vi "FTW-Actor-Destroy.vi"(0 "FTW Actor Instance":refnum<class "FTW-ActorInstance.lvclass">, 11 "error in":errorcluster) -> (15 "error out":errorcluster)   [LabVIEW 2012, in "FTW-Actor.lvlib" / "FTW-ActorInstance.lvclass"]
uses:
  FTW-ActorInstance.lvclass
  JobSequencer/FTW-JobSequencer.lvclass
  EventLogger/FTW-Logger.lvclass
  Endpoint/FTW-Endpoint.lvclass
panel:
  # "Inputs"
  # "Outputs"
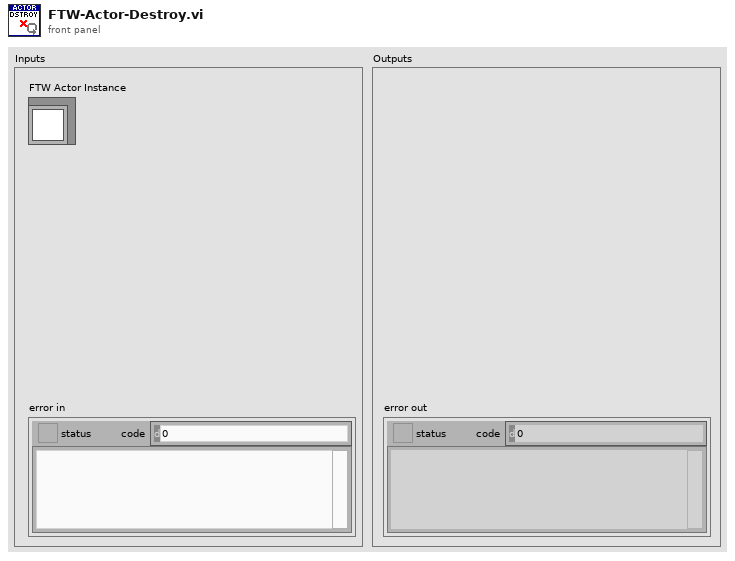
[diagram p1: front panel]
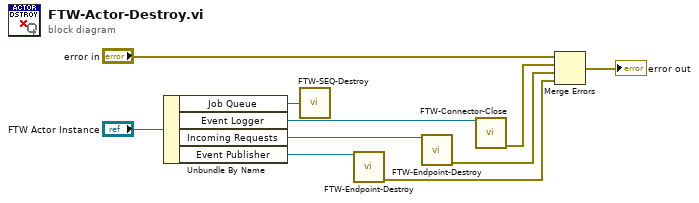
[diagram p0: block diagram]
diagram:
  n1 = Unbundle By Name("FTW Actor Instance") -> ("Job Queue"=w7:refnum<class "FTW-JobSequencer.lvclass">, "Event Logger"=w2:refnum<class "FTW-Logger.lvclass">, "Incoming Requests"=w5:refnum<class "FTW-Endpoint.lvclass">, "Event Publisher"=w4:refnum<class "FTW-Endpoint.lvclass">)
  n2 = call "FTW-SEQ-Destroy.vi"("FTW Job Sequencer"=w7) -> ()  [unwired: 1 in]
  n3 = call-dynamic "FTW-Endpoint-Destroy.vi"("FTW Socket"=w4) -> ("error out"=w3:errorcluster)  [unwired: 14 in]
  n4 = call-dynamic "FTW-Endpoint-Destroy.vi"("FTW Socket"=w5) -> ("error out"=w6:errorcluster)  [unwired: 14 in]
  n5 = call-dynamic "FTW-Connector-Close.vi"("FTW Actor Connector"=w2) -> ("error out"=w1:errorcluster)  [unwired: 14 in]
  n6 = Merge Errors("error in", w1, w6, w3) -> (→"error out":errorcluster)
